vi "Set Variable Values.vi"(8 "error in (no error)":errorcluster, 9 "varValues":dbl[](array[numeric]) format="%#_13g", 10 "varNames":string[](array[string]), 11 "muExpr in":refnum<class "mupExpr.lvclass">) -> (0 "error out":errorcluster, 3 "muExpr out":refnum<class "mupExpr.lvclass">)   [LabVIEW 2015, in "mupExpr.lvclass"]
uses:
  mupExpr.lvclass
  mupExpr.lvclass/mupExpr.ctl
  mupLib/mupSetVarValue.vi
  <vilib>/Utility/error.llb/Error Cluster From Error Code.vi
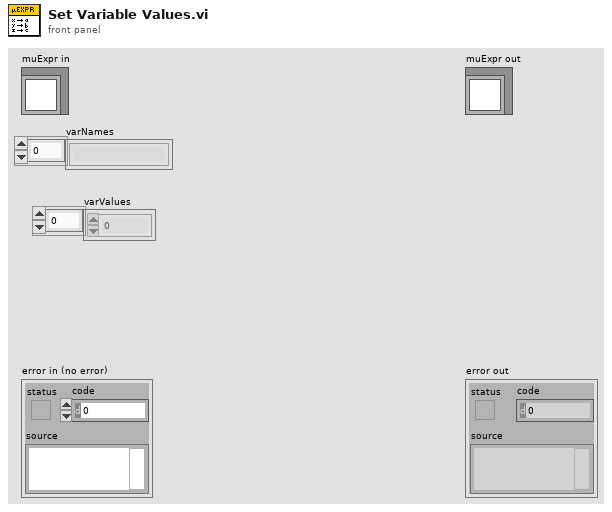
[diagram p1: front panel]
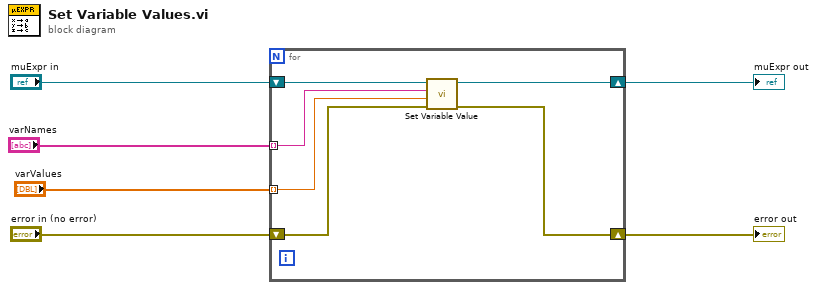
[diagram p0: block diagram]
diagram:
  n1 = for {
    shift-right: [w11] -> w3
    shift-left: "muExpr in" -> [w12]
    tunnel: "varNames" -> [w10] mode=indexing
    tunnel: "varValues" -> [w9] mode=indexing
    shift-right: [w7] -> w5
    shift-left: "error in (no error)" -> [w8]
    n2 = call "Set Variable Value.vi"("error in (no error)"=w8, "varValue"=w9, "varName"=w10, "muExpr in"=w12) -> ("error out"=w7:errorcluster, "muExpr out"=w11:refnum<class "mupExpr.lvclass">)  [unwired: 6 in]
  }
  "error out" <- w5
  "muExpr out" <- w3
